vi "Calculate Curved Motion.vi"(5 "orientation":enum16{"cw", "ccw"}(ring), 6 "Points per revolution":u32=500, 7 "Radius (mm)":dbl, 8 "error in (no error)":errorcluster, 9 "Speed (mm/s)":dbl, 10 "Destination (mm)":refnum<class "Vec3d.lvclass">, 11 "Origin (mm)":refnum<class "Vec3d.lvclass">) -> (0 "error out":errorcluster, 1 "Times (ms)":dbl[](array[numeric]), 2 "Speeds (mm/s)":refnum<class "Vec3d.lvclass">[](array[class]), 3 "Coordinates (mm)":refnum<class "Vec3d.lvclass">[](array[class]))   [LabVIEW 2024]
uses:
  Vec3d Class/Vec3d.lvclass
panel:
  # "Gives output appropriate\nfor feeding to MoveCvt"
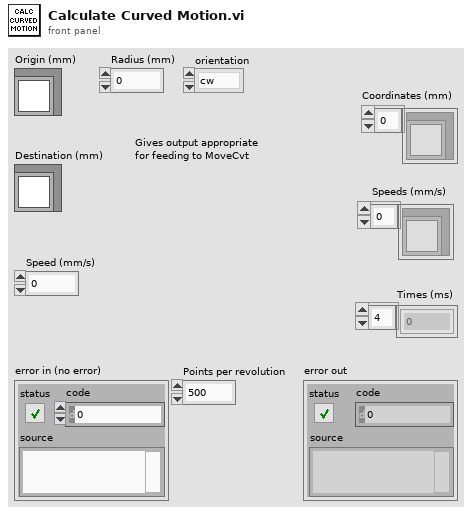
[diagram p1: front panel]
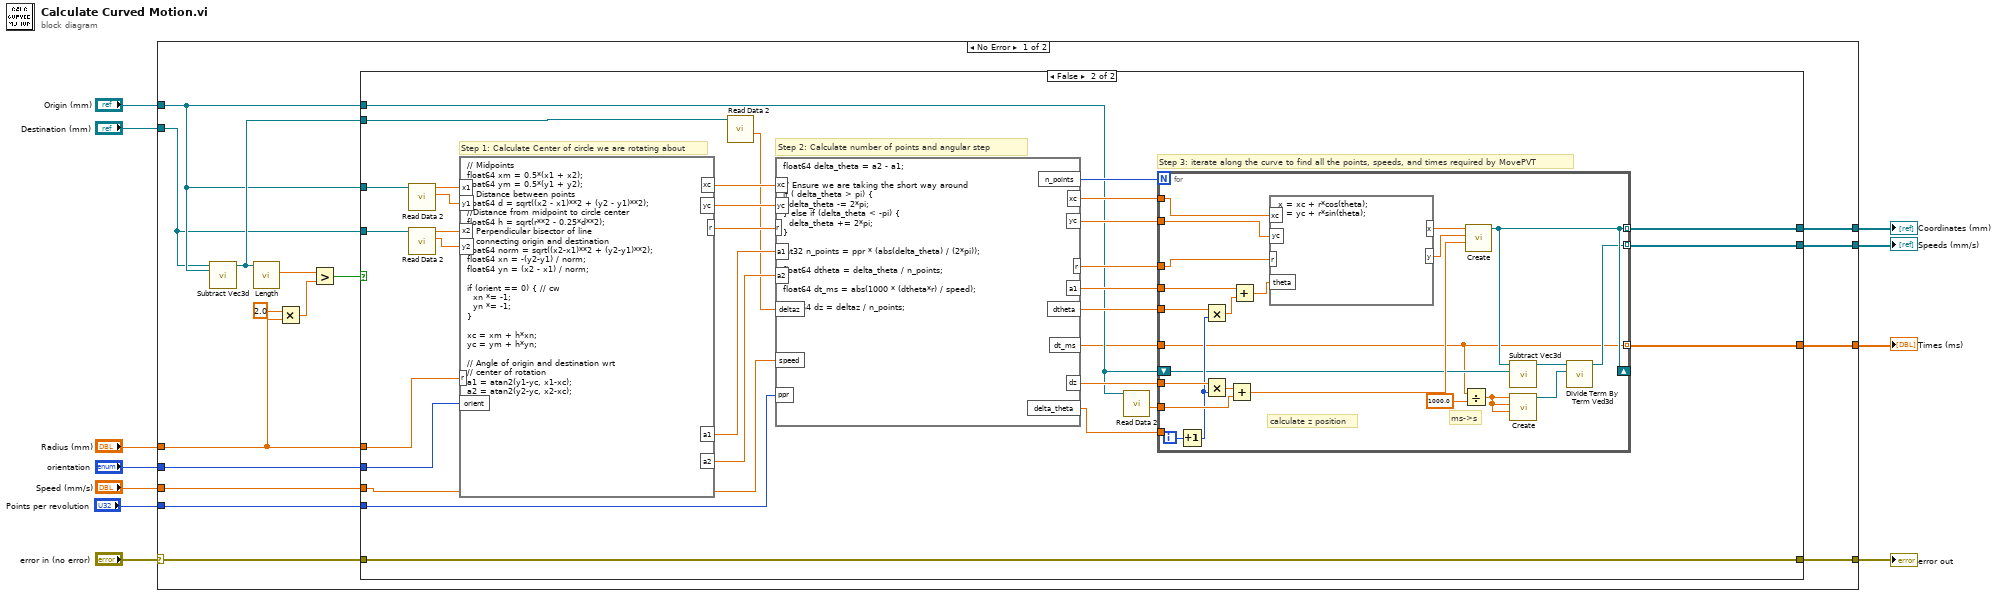
[diagram p0: block diagram]
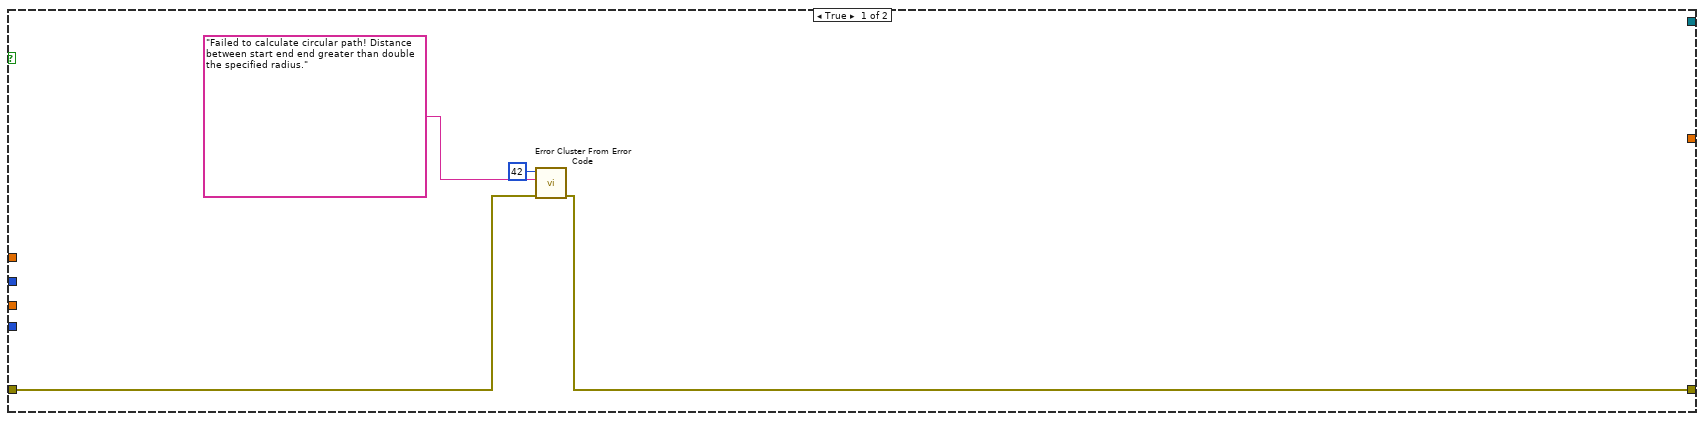
[diagram p2: hidden frame]
diagram:
  n1 = case shown="No Error" "error in (no error)" {
    selector: "error in (no error)" -> [w21 w87]
    tunnel: [w20 w87] -> w10
    tunnel: "Origin (mm)" -> [w16 _]
    tunnel: "Destination (mm)" -> [w15 _]
    tunnel: "Radius (mm)" -> [w26 _]
    tunnel: "orientation" -> [w27 _]
    tunnel: "Speed (mm/s)" -> [w19 _]
    tunnel: "Points per revolution" -> [w18 _]
    tunnel: [w14 _] -> w3
    tunnel: [w13 _] -> w2
    tunnel: [w12 _] -> w1
    frame No Error {
      n2 = call "Subtract Vec3d.vi"("Vec3d in 2"=w16, "Vec3d in 1"=w15) -> ("Vec3d Class out"=w17:refnum<class "Vec3d.lvclass">)  [unwired: 8 in, 1 out]
      n3 = call-dynamic "Length.vi"("Vec3d in"=w17) -> ("Length"=w24:dbl)  [unwired: 8 in, 2 out]
      n4 = Multiply(x=2.0, y=w26) -> (x*y=w23:dbl)
      n5 = Greater?(x=w24, y=w23) -> (0:w22:bool)
      n6 = case shown="False" w22 {
        tunnel: w15 -> [_ w63]
        tunnel: w16 -> [_ w62]
        tunnel: w26 -> [_ w57]
        tunnel: w27 -> [_ w56]
        tunnel: w21 -> [w31 w50]
        tunnel: [w30 w50] -> w20
        tunnel: w19 -> [_ w42]
        tunnel: w18 -> [_ w49]
        tunnel: w16 -> [_ w38]
        tunnel: w17 -> [_ w41]
        tunnel: [_ w35] -> w14
        tunnel: [_ w34] -> w13
        tunnel: [_ w33] -> w12
        frame True {
          n7 = call <vilib>:"Error Cluster From Error Code.vi"("error in (no error)"=w31, "error message (\"\")"="Failed to calculate circular path! Distance between start end end greater than double the specified radius." ("error message (\"\")"), "error code (0)"=42) -> ("error out"=w30:errorcluster)  [unwired: 6 in]
        }
        frame False {
          # "Step 3: iterate along the curve to find all the points, speeds, and times required by MovePVT"
          # "Step 2: Calculate number of points and angular step"
          # "Step 1: Calculate Center of circle we are rotating about"
          n8 = call-dynamic "Read Data 2.vi"("Vec3d in"=w62) -> ("Y"=w60:dbl, "X"=w61:dbl)  [unwired: 7 in, 2 out]
          n9 = call-dynamic "Read Data 2.vi"("Vec3d in"=w63) -> ("Y"=w58:dbl, "X"=w59:dbl)  [unwired: 7 in, 2 out]
          n10 = formula code="// Midpoints\nfloat64 xm = 0.5*(x1 + x2);\nfloat64 ym = 0.5*(y1 + y2);\n// Distance between points\nfloat64 d = sqrt((x2 - x1)**2 + (y2 - y1)**2);\n//Distance from midpoint to circle center\nfloat64 h = sqrt(r**2 - 0.25*d**2);\n// Perpendicular bisector of line \n// connecting origin and destination\nfloat64 norm = sqrt((x2-x1)**2 + (y2-y1)**2);\nfloat64 xn = -(y2-y1) / norm;\nfloat64 yn = (x2 - x1) / norm;\n\nif (orient == 0) { // cw\n  xn *= -1;\n  yn *= -1;\n}\n\nxc = xm + h*xn;\nyc = ym + h*yn;\n\n// Angle of origin and destination wrt\n// center of rotation\na1 = atan2(y1-yc, x1-xc);\na2 = atan2(y2-yc, x2-xc);"("x1"=w61, "y1"=w60, "x2"=w59, "y2"=w58, "r"=w57, "orient"=w56) -> ("xc"=w55:dbl, "yc"=w54:dbl, "a1"=w53:dbl, "a2"=w52:dbl, "r"=w51:dbl)
          n11 = call-dynamic "Read Data 2.vi"("Vec3d in"=w41) -> ("Z"=w40:dbl)  [unwired: 7 in, 3 out]
          n12 = formula code="float64 delta_theta = a2 - a1;\n\n// Ensure we are taking the short way around\nif ( delta_theta > pi) {\n  delta_theta -= 2*pi;\n} else if (delta_theta < -pi) {\n  delta_theta += 2*pi;\n}\n\nint32 n_points = ppr * (abs(delta_theta) / (2*pi));\n\nfloat64 dtheta = delta_theta / n_points;\n\nfloat64 dt_ms = abs(1000 * (dtheta*r) / speed);\n\nfloat64 dz = deltaz / n_points;"("xc"=w55, "yc"=w54, "a1"=w53, "a2"=w52, "r"=w51, "ppr"=w49, "speed"=w42, "deltaz"=w40) -> ("n_points"=w48:i32, "dtheta"=w43:dbl, "r"=w44:dbl, "xc"=w47:dbl, "yc"=w46:dbl, "a1"=w45:dbl, "dz"=w39:dbl, "dt_ms"=w36:dbl, "delta_theta"=w32:dbl)
          n13 = call-dynamic "Read Data 2.vi"("Vec3d in"=w38) -> ("Z"=w37:dbl)  [unwired: 7 in, 3 out]
          n14 = for {
            N: w48 -> [_]
            shift-right: [w70] -> _
            shift-left: w38 -> [w71]
            tunnel: w47 -> [w76]
            tunnel: w46 -> [w75]
            tunnel: w45 -> [w79]
            tunnel: w44 -> [w77]
            tunnel: w43 -> [w81]
            tunnel: w39 -> [w85]
            tunnel: w37 -> [w83]
            tunnel: w36 -> [w66]
            tunnel: [w70] -> w35 mode=indexing
            tunnel: [w67] -> w34 mode=indexing
            tunnel: [w66] -> w33 mode=indexing
            tunnel: w32 -> [_]
            i -> [w86]
            # "ms->s"
            # "calculate z position"
            n15 = Increment(x=w86) -> (x+1=w82:i32)
            n16 = Multiply(x=w81, y=w82) -> (x*y=w80:dbl)
            n17 = Multiply(x=w85, y=w82) -> (x*y=w84:dbl)
            n18 = Add(x=w84, y=w83) -> (x+y=w72:dbl)
            n19 = Add(x=w79, y=w80) -> (x+y=w78:dbl)
            n20 = formula code="x = xc + r*cos(theta);\ny = yc + r*sin(theta);"("xc"=w76, "yc"=w75, "r"=w77, "theta"=w78) -> ("x"=w74:dbl, "y"=w73:dbl)
            n21 = Divide(x=w66, y=1000.0) -> (x/y=w65:dbl)
            n22 = call "Create.vi"("Z"=w72, "Y"=w73, "X"=w74) -> ("Vec3d Class out"=w70:refnum<class "Vec3d.lvclass">)  [unwired: 7 in, 1 out]
            n23 = call "Subtract Vec3d.vi"("Vec3d in 2"=w71, "Vec3d in 1"=w70) -> ("Vec3d Class out"=w69:refnum<class "Vec3d.lvclass">)  [unwired: 8 in, 1 out]
            n24 = call "Create.vi"("Z"=w65, "Y"=w65, "X"=w65) -> ("Vec3d Class out"=w68:refnum<class "Vec3d.lvclass">)  [unwired: 7 in, 1 out]
            n25 = call-dynamic "Divide Term By Term Ved3d.vi"("Vec3d in 2"=w68, "Vec3d in 1"=w69) -> ("Vec3d Class out"=w67:refnum<class "Vec3d.lvclass">)  [unwired: 8 in, 1 out]
          }
        }
      }
    }
    frame Error {
    }
  }
  "error out" <- w10
  "Coordinates (mm)" <- w3
  "Times (ms)" <- w1
  "Speeds (mm/s)" <- w2
